vi "Array Dot Product.vi"(0 "array a":dbl[](array[numeric]), 2 "array b":dbl[](array[numeric])) -> (7 "a . b":dbl)   [LabVIEW 2014]
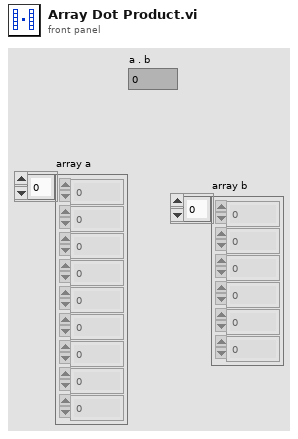
[diagram p1: front panel]
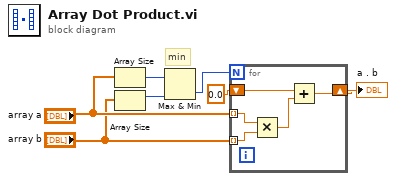
[diagram p0: block diagram]
diagram:
  # "min"
  n1 = Array Size(array="array a") -> (size(s)=w3:i32)
  n2 = Array Size(array="array b") -> (size(s)=w2:i32)
  n3 = Max & Min(x=w3, y=w2) -> (min(x,y)=w1:i32)  [unwired: 1 out]
  n4 = for {
    N: w1 -> [_]
    tunnel: "array a" -> [w11] mode=indexing
    shift-right: [w10] -> w7
    shift-left: 0.0 -> [w9]
    tunnel: "array b" -> [w12] mode=indexing
    n5 = Multiply(x=w11, y=w12) -> (x*y=w8:dbl)
    n6 = Add(x=w9, y=w8) -> (x+y=w10:dbl)
  }
  "a . b" <- w7
